vi "Analog Continous Input.vi"() -> ()   [LabVIEW 2009, in "MicroDAQ.lvlib"]
doc: "This example demonstrates how to continuously acquire buffered analog measurements using a microDAQ device.\n\nFor instructions on how to connect your signals to the DAQ device, refer to your device documentation."
uses:
  <instrlib>/MicroDAQ/MicroDAQ.lvlib
  <instrlib>/MicroDAQ/Tools/Analog input type enum.ctl
  <instrlib>/MicroDAQ/Tools/Analog input Channel enum.ctl
  <instrlib>/MicroDAQ/Tools/Analo Range Enum.ctl
  <instrlib>/MicroDAQ/Tools/Encoder type.ctl
  <instrlib>/MicroDAQ/Tools/Trigger Encoder condition enum.ctl
  <instrlib>/MicroDAQ/Channel/Analog Input/AI Configure Channel.vi
  <instrlib>/MicroDAQ/Channel/Analog Input/Triggering DIO state.vi
  <instrlib>/MicroDAQ/Channel/Analog Input/Triggering DIO Pattern.vi
  <instrlib>/MicroDAQ/Channel/Analog Input/Triggering Encoder.vi
  <instrlib>/MicroDAQ/Channel/Analog Input/Analog Input.lvclass
  <instrlib>/MicroDAQ/Channel/Analog Input/Read NChan NSamp 2D SGL.vi
panel:
  in  "Triggering":T1(tab)
  in  "Digital input pin":u8
  in  "Level":bool=TRUE
  in  "Pattern":string
  in  "Condition":T2
  in  "Position":i32
  in  "Channel":T3 items=["ENC1"=1, "ENC2"=2]
  in  "Read samples per channel":i32=100
  in  "Stop":bool
  out "Waveform Graph":dbl[][](graph)
  in  "Sample Rate [Hz]":dbl=1000.0 format="%#_13g"
  in  "Ranges":T4[](array[typedef])=[enum."±10V"]
  in  "IP address":string="10.10.1.1"
  in  "Physical channels":T5[](array[typedef])=[enum."AI1"]
  in  "Number of samples per channel":i32=-1
  in  "Input terminals configurations":T6[](array[typedef])=[enum."Single-ended"]
  # "Device settings"
  # "Read Settings"
  # "Channel Settings"
  # "Input"
  # "Mode and Timing Settings"
  # "* \"-1\" value or continous execution"
  # "Tip: x->ignored, 1->HI, 0->LOW\nexampe: 11xxxxxx\nmore info in Triggering VI help"
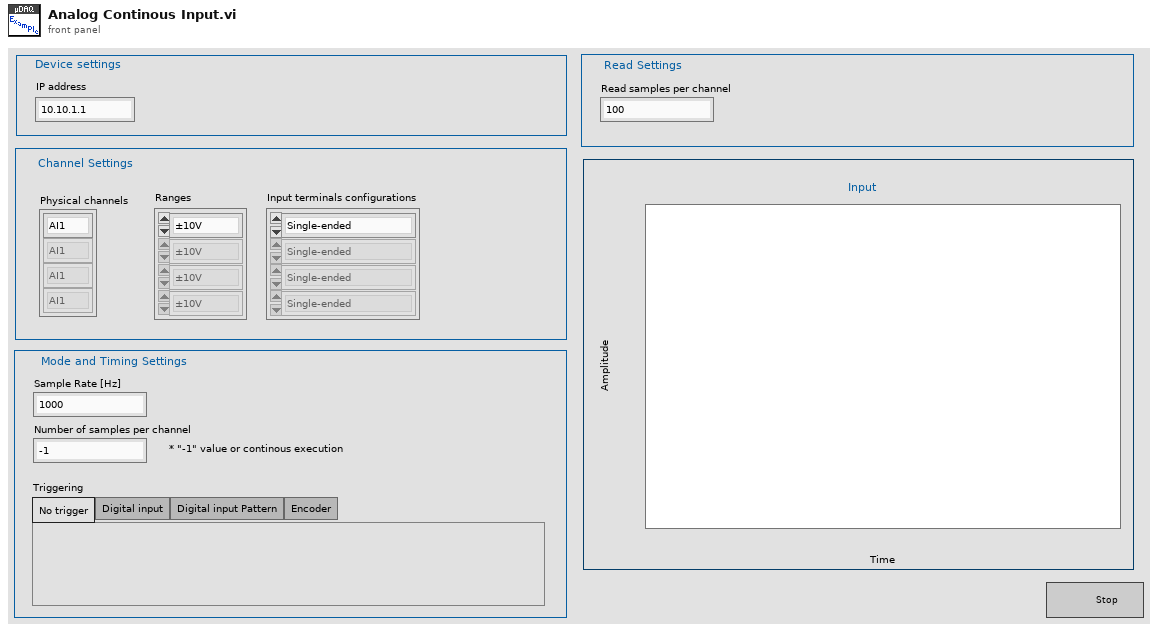
[diagram p1: front panel]
types:
  T1 = enum32{"No trigger", "Digital input", "Digital input Pattern", "Encoder"}
  T2 = typedef "MicroDAQ.lvlib/Trigger Encoder condition enum.ctl" = enum16{"Lower then", "Greater then"}
  T3 = typedef "MicroDAQ.lvlib/Encoder type.ctl" = u8
  T4 = typedef "MicroDAQ.lvlib/Analo Range Enum.ctl" = enum16{"±10V", "0-10V", "±5V", "0-5V", "±5.12V", "±2.56V", "±2.5V", "±2V", "±1.24V", "±0.64V"}
  T5 = typedef "MicroDAQ.lvlib/Analog input Channel enum.ctl" = enum16{"None", "AI1", "AI2", "AI3", "AI4", "AI5", "AI6", "AI7", "AI8", "AI9", "AI10", "AI11", "AI12", "AI13", "AI14", "AI15", "AI16"}
  T6 = typedef "MicroDAQ.lvlib/Analog input type enum.ctl" = enum16{"Single-ended", "Differential"}
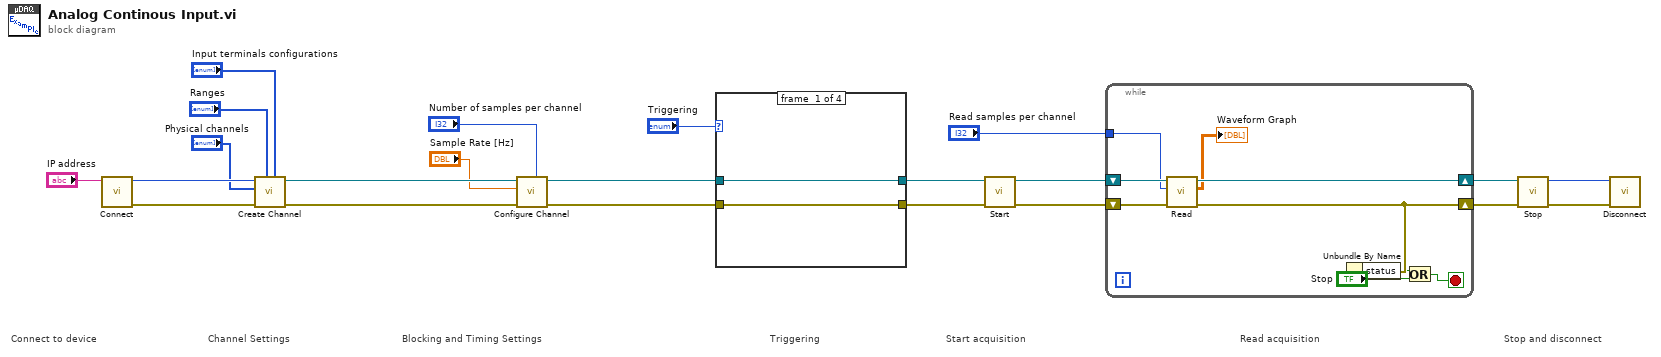
[diagram p0: block diagram]
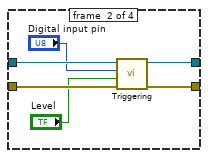
[diagram p2: hidden frame]
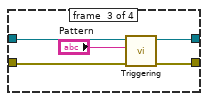
[diagram p3: hidden frame]
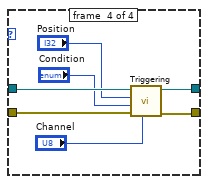
[diagram p4: hidden frame]
diagram:
  # "Triggering"
  # "Stop and disconnect"
  # "Connect to device"
  # "Read acquisition"
  # "Start acquisition"
  # "Blocking and Timing Settings"
  # "Channel Settings"
  n1 = call <instrlib>:"Connect.vi"("IP address"="IP address") -> ("error out"=w21:errorcluster, "connection ID"=w22:i32)  [unwired: 9 in]
  n2 = call-poly <instrlib>:"Create Channel.vi"("Input terminals configurations"="Input terminals configurations", "Ranges"="Ranges", "error in (no error)"=w21, "Phisical channels"="Physical channels", "connection ID"=w22) -> ("error out"=w19:errorcluster, "Task Out"=w20:refnum<class "Analog Input.lvclass">)  [unwired: 5 in]
  n3 = call-poly <instrlib>:"Configure Channel.vi"("Samples per channel"="Number of samples per channel", "error in (no error)"=w19, "Sampe Rate"="Sample Rate [Hz]", "MicroDAQ.lvlib:Analog Input.lvclass"=w20) -> ("error out"=w2:errorcluster, "MicroDAQ.lvlib:Analog Input.lvclass out"=w4:refnum<class "Analog Input.lvclass">)  [unwired: 6 in]
  n4 = case shown="\"Encoder\"" "Triggering" {
    tunnel: w4 -> [w24 w30 w35 w41]
    tunnel: [w24 w29 w32 w42] -> w3
    tunnel: w2 -> [w23 w28 w34 w40]
    tunnel: [w23 w27 w33 w39] -> w1
    frame #0 {
    }
    frame #1 {
      n5 = call-poly <instrlib>:"Triggering.vi"("error in (no error)"=w28, "level"="Level", "pin"="Digital input pin", "MicroDAQ.lvlib:Analog Input.lvclass"=w30) -> ("error out"=w27:errorcluster, "MicroDAQ.lvlib:Analog Input.lvclass out"=w29:refnum<class "Analog Input.lvclass">)  [unwired: 6 in]
    }
    frame #2 {
      n6 = call-poly <instrlib>:"Triggering.vi"("error in (no error)"=w34, "pattern"="Pattern", "MicroDAQ.lvlib:Analog Input.lvclass"=w35) -> ("error out"=w33:errorcluster, "MicroDAQ.lvlib:Analog Input.lvclass out"=w32:refnum<class "Analog Input.lvclass">)  [unwired: 7 in]
    }
    frame #3 {
      n7 = call-poly <instrlib>:"Triggering.vi"("Channel (1|2)"="Channel", "error in (no error)"=w40, "condition"="Condition", "position"="Position", "MicroDAQ.lvlib:Analog Input.lvclass"=w41) -> ("error out"=w39:errorcluster, "MicroDAQ.lvlib:Analog Input.lvclass out"=w42:refnum<class "Analog Input.lvclass">)  [unwired: 5 in]
    }
  }
  n8 = call-dynamic "Start.vi"("error in (no error)"=w1, "Analog Input in"=w3) -> ("error out"=w17:errorcluster, "Analog Input out"=w18:refnum<class "Analog Input.lvclass">)  [unwired: 8 in]
  n9 = while {
    tunnel: "Read samples per channel" -> [w48]
    shift-right: [w49] -> w16
    shift-left: w18 -> [w51]
    shift-right: [w45] -> w15
    shift-left: w17 -> [w50]
    stop <- w44 stop-if-true
    n10 = call-poly <instrlib>:"Read.vi"("error in (no error)"=w50, "number of samples per channel"=w48, "MicroDAQ.lvlib:Analog Input.lvclass"=w51) -> ("error out"=w45:errorcluster, "Values"=→"Waveform Graph":dbl[][], "MicroDAQ.lvlib:Analog Input.lvclass out"=w49:refnum<class "Analog Input.lvclass">)  [unwired: 5 in, 1 out]
    n11 = Unbundle By Name(w45) -> ("status"=w43:bool)
    n12 = Or(x=w43, y="Stop") -> (x .or. y?=w44:bool)
  }
  n13 = call-dynamic "Stop.vi"("error in (no error)"=w15, "Analog Input in"=w16) -> ("error out"=w13:errorcluster, "connection ID"=w14:i32)  [unwired: 8 in]
  n14 = call <instrlib>:"Disconnect.vi"("error in (no error)"=w13, "connection ID"=w14) -> ()  [unwired: 9 in, 1 out]
